vi "Button Enabled.vi"(6 "error in":errorcluster, 9 "button refnum":refnum<vi>) -> (0 "error out":errorcluster, 3 "button refnum dup":refnum<vi>)   [LabVIEW 2020]
doc: "This function sets the button state to \"Enabled\"."
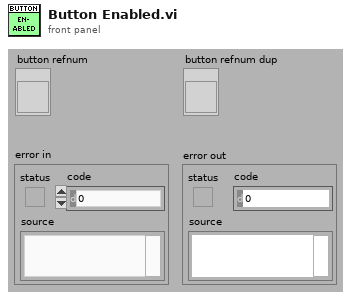
[diagram p1: front panel]
types:
  T1 = enum8{"Enabled", "Disabled", "Disabled and Grayed Out"}
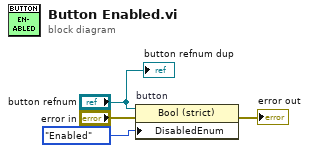
[diagram p0: block diagram]
diagram:
  n1 = property on="button" class="Bool (strict)"(reference="button refnum", error in="error in", "DisabledEnum"=T1."Enabled" ("Disabled")) -> (error out=→"error out":errorcluster)  [unwired: 1 out]
  "button refnum dup" <- "button refnum"
